vi "run_tests.vi"() -> ()   [LabVIEW 2020]
uses:
  <vilib>/addons/_JKI Toolkits/Caraya/run-tests/Run Test (Scalar Path).vi
  <vilib>/addons/_JKI Toolkits/Caraya/Caraya.lvlib
panel:
  in  "Interactive (T)":bool=TRUE
  out "error out":errorcluster
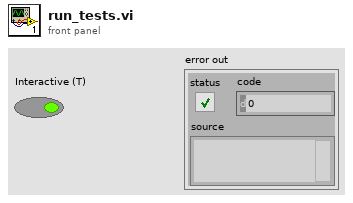
[diagram p1: front panel]
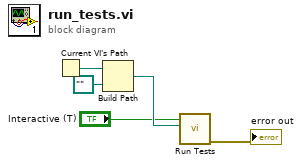
[diagram p0: block diagram]
diagram:
  n1 = Current VI's Path() -> (path=w5:path)
  n2 = Build Path(base path=w5, name or relative path=path "..") -> (appended path=w3:path)
  n3 = call-poly <vilib>:"Run Tests.vi"("Test Path"=w3, "Interactive (T)"="Interactive (T)") -> ("error out"=→"error out":errorcluster)  [unwired: 8 in, 1 out]
